vi "ExecuteMenuCommand.vi"(0 "reference":refnum<class "ClassNode.lvclass">, 1 "Command":string, 5 "error in (no error)":errorcluster) -> (14 "reference out":refnum<class "ClassNode.lvclass">, 15 "EditorAction":T3, 16 "FlattenCommandSettings":T1, 19 "error out":errorcluster)   [LabVIEW 2020, in "ClassNode.lvclass"]
uses:
  <resource>/Framework/Providers/Open_GDS/UML/ClassNode_class/ClassNode.lvclass
  <resource>/Framework/Providers/Open_GDS/UML/UMLEditor/UMLEditor EditorActionType.ctl
  <resource>/Framework/Providers/Open_GDS/UML/UMLEditor/UMLEditor FlattenCommandType.ctl
  <resource>/Framework/Providers/Open_GDS/UML/UMLEditor/UMLEditor ExecuteCommandType.ctl
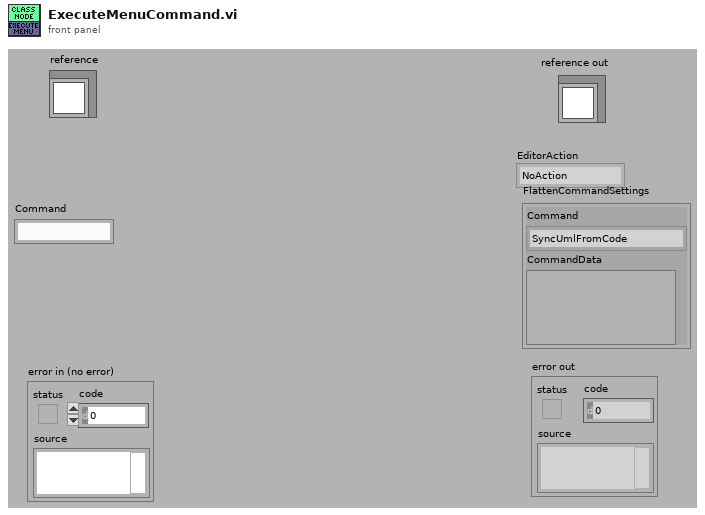
[diagram p1: front panel]
types:
  T1 = typedef "UMLEditor FlattenCommandType.ctl" = cluster{"Command":T2, "CommandData":variant}
  T2 = typedef "UMLEditor ExecuteCommandType.ctl" = enum16{"SyncUmlFromCode", "SyncCodeFromUML", "OpenClass", "OpenFile", "CreateClass", "CreateVI", "OpenClassAttribute", "LocateInProject", "GraphExecute"}
  T3 = typedef "UMLEditor EditorActionType.ctl" = enum16{"NoAction", "Repaint", "ExecuteCommand"}
  T4 = typedef "ClassNode.lvclass/ObjectAttributes.ctl" = cluster{"midHeight":dbl, "botHeight":dbl, "name":refnum<class "MultiLineString.lvclass">, "attributes":refnum<class "MultiLineString.lvclass">, "methods":refnum<class "MultiLineString.lvclass">, "DEFAULT_COMPARTMENT_HEIGHT":i32, "DEFAULT_WIDTH":i32, "DEFAULT_HEIGHT":i32, "showMethods":bool, "showAttributes":bool, "ClassPath":path}
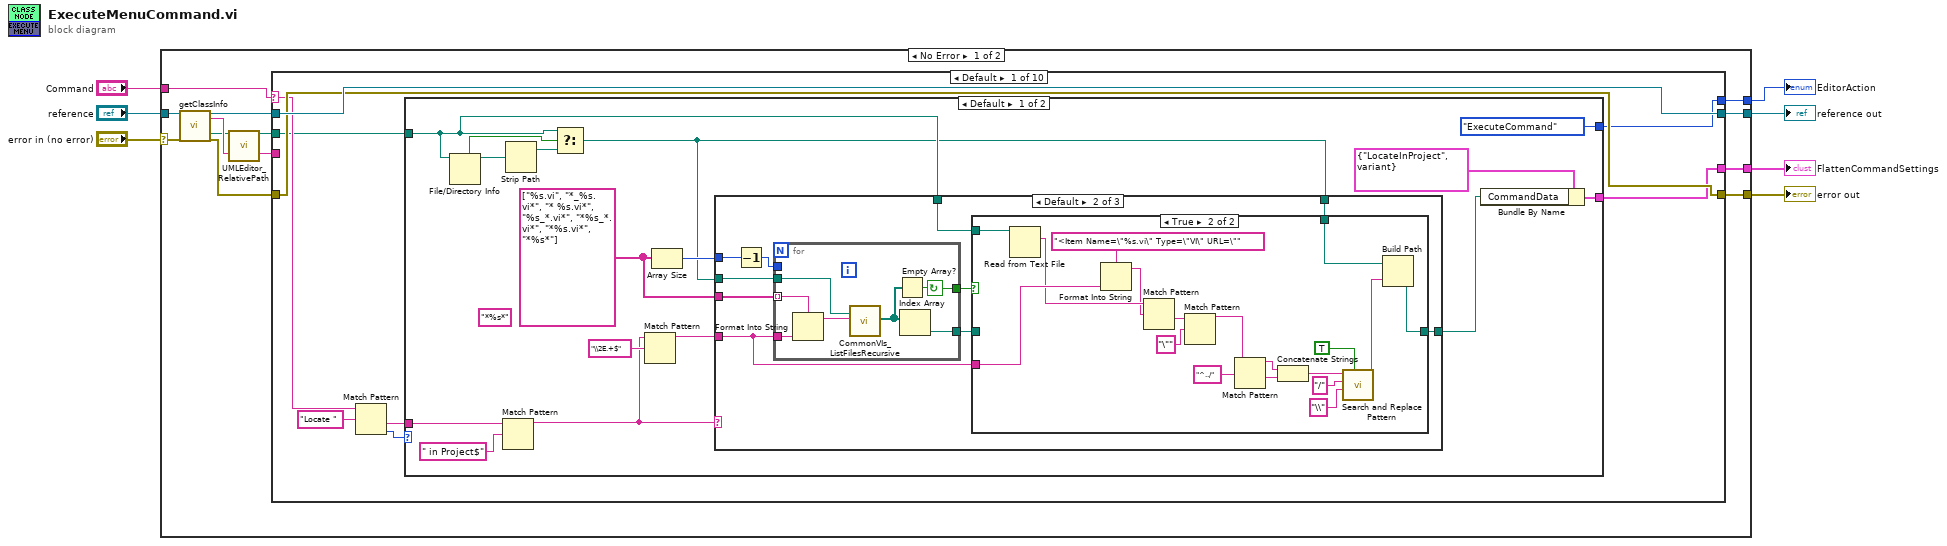
[diagram p0: block diagram]
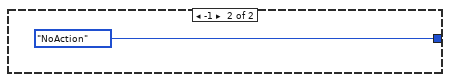
[diagram p5: hidden frame]
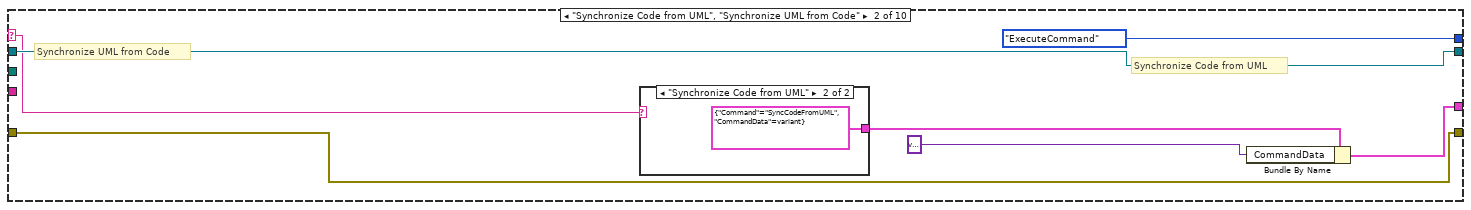
[diagram p6: hidden frame]
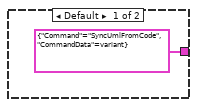
[diagram p7: hidden frame]
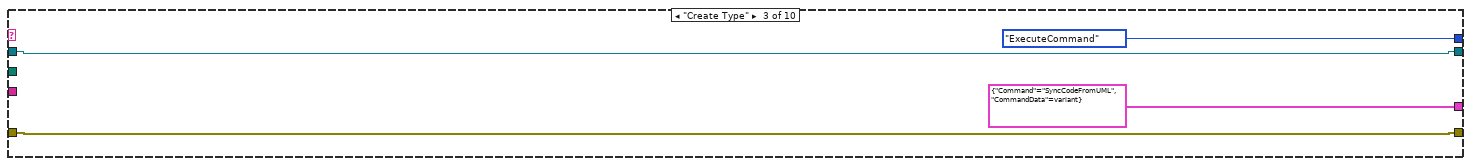
[diagram p8: hidden frame]
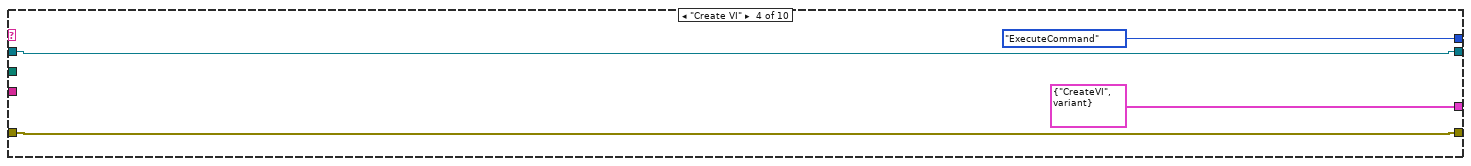
[diagram p9: hidden frame]
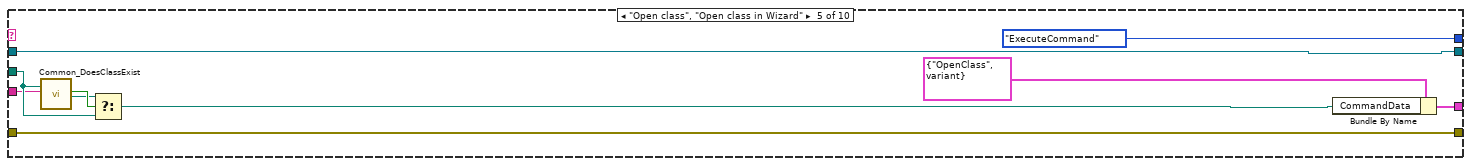
[diagram p10: hidden frame]
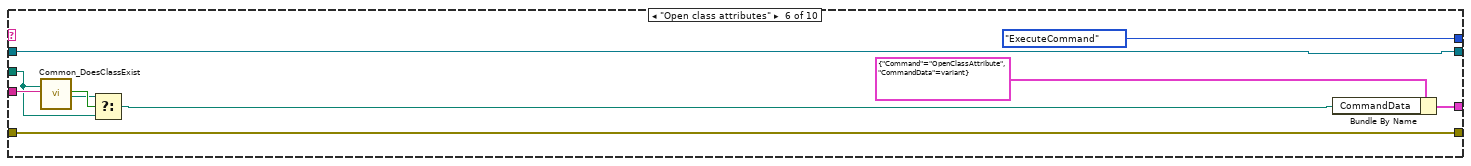
[diagram p11: hidden frame]
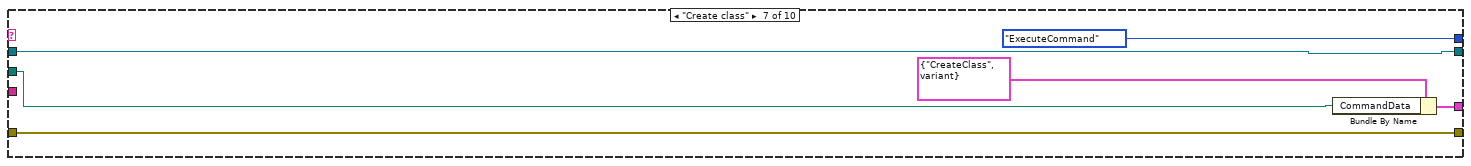
[diagram p12: hidden frame]
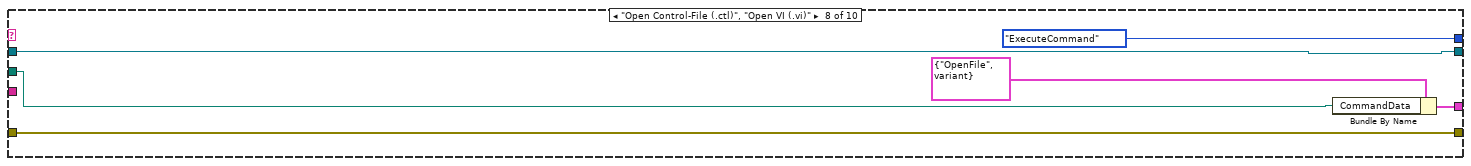
[diagram p13: hidden frame]
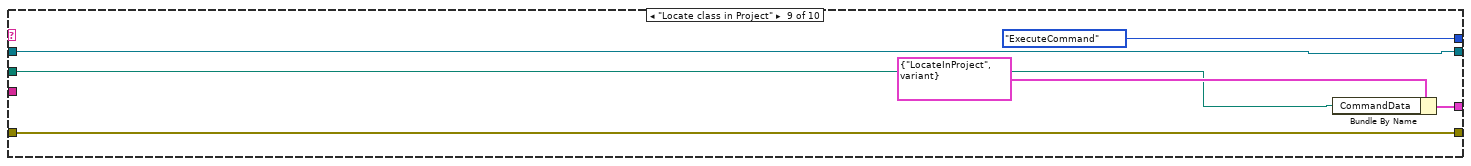
[diagram p14: hidden frame]
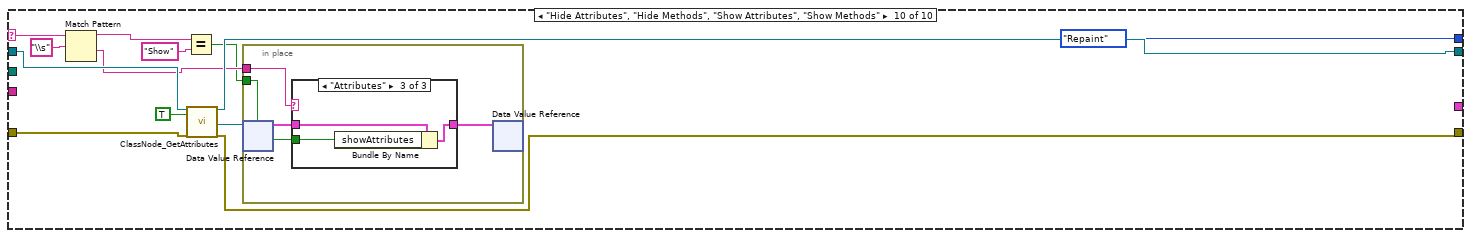
[diagram p15: hidden frame]
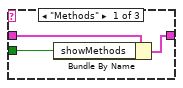
[diagram p16: hidden frame]
diagram:
  n1 = case shown="No Error" "error in (no error)" {
    selector: "error in (no error)" -> [w12 w162]
    tunnel: "reference" -> [w14 w163]
    tunnel: [w17 w162] -> w5
    tunnel: [w18 w163] -> w4
    tunnel: "Command" -> [w19 _]
    tunnel: [w16 _] -> w2
    tunnel: [w15 _] -> w1
    frame No Error {
      n2 = call-dynamic "getClassInfo.vi"("reference"=w14, "error in (no error)"=w12) -> ("reference out"=w13:refnum<class "ClassNode.lvclass">, "className"=w10:string, "ClassPath"=w9:path, "error out"=w11:errorcluster)  [unwired: 8 in, 6 out]
      n3 = call <resource>:"UMLEditor_RelativePath.vi"("Path In"=w9) -> ("ConvertToAbsolutePath(If possible)"=w8:path)  [unwired: 1 in, 17 out]
      n4 = case shown="Default" w19 {
        selector: w19 -> [w25 w83 _ _ _ _ _ _ _ w145]
        tunnel: w11 -> [w27 w87 w92 w96 w107 w110 w123 w129 w135 w147]
        tunnel: w13 -> [w28 w88 w93 w97 w108 w118 w124 w130 w136 w149]
        tunnel: [w28 w88 w93 w97 w108 w118 w124 w130 w136 w148] -> w18
        tunnel: [w27 w87 w92 w96 w107 w110 w123 w129 w135 w146] -> w17
        tunnel: [w26 UMLEditor_EditorActionType."ExecuteCommand" ("EditorAction") UMLEditor_EditorActionType."ExecuteCommand" ("EditorAction") UMLEditor_EditorActionType."ExecuteCommand" ("EditorAction") UMLEditor_EditorActionType."ExecuteCommand" ("EditorAction") UMLEditor_EditorActionType."ExecuteCommand" ("EditorAction") UMLEditor_EditorActionType."ExecuteCommand" ("EditorAction") UMLEditor_EditorActionType."ExecuteCommand" ("EditorAction") UMLEditor_EditorActionType."ExecuteCommand" ("EditorAction") UMLEditor_EditorActionType."Repaint" ("EditorAction")] -> w16
        tunnel: [w21 w85 T1 {"Command"=enum."SyncCodeFromUML", "CommandData"=variant} ("FlattenCommandSettings") T1 {"Command"=enum."CreateVI", "CommandData"=variant} ("FlattenCommandSettings") w105 w116 w121 w127 w133 _] -> w15
        tunnel: w8 -> [w20 _ _ _ w101 w111 w120 w126 w132 _]
        tunnel: w10 -> [_ _ _ _ w100 w112 _ _ _ _]
        frame Default {
          n5 = Match Pattern(string=w25, regular expression="Locate ") -> (after substring=w22:string, offset past match=w23:i32)  [unwired: 1 in, 2 out]
          n6 = case shown="Default" w23 {
            tunnel: [UMLEditor_EditorActionType."ExecuteCommand" ("EditorAction") UMLEditor_EditorActionType."NoAction" ("EditorAction")] -> w26
            tunnel: w22 -> [w44 _]
            tunnel: [w40 _] -> w21
            tunnel: w20 -> [w30 _]
            frame Default {
              (unwired) "*%s*" ("format string")
              w36 = string[] ["%s.vi", "*_%s.vi*", "* %s.vi*", "%s_*.vi*", "*%s_*.vi*", "*%s.vi*", "*%s*"]
              n7 = File/Directory Info(path=w30) -> (path out=w34:path, directory=w38:bool)  [unwired: 1 in, 5 out]
              n8 = Match Pattern(string=w44, regular expression=" in Project$") -> (before substring=w32:string)  [unwired: 1 in, 3 out]
              n9 = Strip Path(path=w34) -> (stripped path=w33:path)  [unwired: 1 out]
              n10 = Select(t=w30, s=w38, f=w33) -> (s? t:f=w29:path)
              n11 = Match Pattern(string=w32, regular expression="\\2E.+$") -> (before substring=w37:string)  [unwired: 4 out]
              n12 = Array Size(array=w36) -> (size(s)=w35:i32)
              n13 = case shown="Default" w32 {
                tunnel: [_ w48 w81] -> w31
                tunnel: w29 -> [_ w54 _]
                tunnel: w36 -> [_ w53 _]
                tunnel: w37 -> [_ w46 _]
                tunnel: w35 -> [_ w52 _]
                tunnel: w30 -> [_ w47 w81]
                tunnel: w29 -> [_ w45 _]
                frame "" {
                }
                frame Default {
                  n14 = Decrement(x=w52) -> (x-1=w51:i32)
                  n15 = for {
                    tunnel: w54 -> [w61]
                    tunnel: w53 -> [w60] mode=indexing
                    tunnel: w46 -> [w59]
                    tunnel: [w58] -> w49
                    tunnel: w51 -> [_]
                    tunnel: [w55] -> w50
                    stop <- w55 continue-if-true
                    n16 = Format Into String(format string=w60, w59) -> (resulting string=w56:string)  [unwired: 2 in, 1 out]
                    n17 = call <resource>:"CommonVIs_ListFilesRecursive.vi"("directory path"=w61, "FileSearchPattern"=w56) -> ("Files"=w57:path[])  [unwired: 4 in, 13 out]
                    n18 = Empty Array?(array=w57) -> (empty?=w55:bool)
                    n19 = Index Array(array=w57) -> (element=w58:path)  [unwired: 1 in]
                  }
                  n20 = case shown="True" w50 {
                    tunnel: w49 -> [w62 _]
                    tunnel: [w62 w63] -> w48
                    tunnel: w47 -> [_ w80]
                    tunnel: w46 -> [_ w78]
                    tunnel: w45 -> [_ w73]
                    frame False {
                    }
                    frame True {
                      n21 = Read from Text File(file (use dialog)=w80) -> (text=w77:string)  [unwired: 3 in, 3 out]
                      n22 = Format Into String(format string="<Item Name=\"%s.vi\" Type=\"VI\" URL=\"" ("regular expression"), w78) -> (resulting string=w76:string)  [unwired: 2 in, 1 out]
                      n23 = Match Pattern(string=w77, regular expression=w76) -> (after substring=w75:string)  [unwired: 1 in, 3 out]
                      n24 = Match Pattern(string=w75, regular expression="\"") -> (before substring=w65:string)  [unwired: 1 in, 3 out]
                      n25 = Match Pattern(string=w65, regular expression="^../") -> (before substring=w72:string, after substring=w71:string)  [unwired: 1 in, 2 out]
                      n26 = Concatenate Strings(w72, w71) -> (w70:string)
                      n27 = call <vilib>:"Search and Replace Pattern.vi"("string"=w70, "regular expression (\"\")"="/" ("regular expression (\"\")"), "replace string (\"\")"="\\" ("replace string (\"\")"), "replace all? (F)"=TRUE) -> ("result string"=w64:string)  [unwired: 1 in, 1 out]
                      n28 = Build Path(base path=w73, name or relative path=w64) -> (appended path=w63:path)
                    }
                  }
                }
                frame "item" {
                }
              }
              n29 = Bundle By Name(cluster=T1 {"Command"=enum."LocateInProject", "CommandData"=variant} ("FlattenCommandSettings"), "CommandData"=w31) -> (w40:T1)
            }
            frame -1 {
            }
          }
        }
        frame "Synchronize Code from UML", "Synchronize UML from Code" {
          # "Synchronize Code from UML"
          # "Synchronize UML from Code"
          n30 = case shown="\"Synchronize Code from UML\"" w83 {
            tunnel: [T1 {"Command"=enum."SyncUmlFromCode", "CommandData"=variant} ("FlattenCommandSettings") T1 {"Command"=enum."SyncCodeFromUML", "CommandData"=variant} ("FlattenCommandSettings")] -> w86
            frame Default {
            }
            frame "Synchronize Code from UML" {
            }
          }
          n31 = Bundle By Name(cluster=w86, "CommandData"=variant) -> (w85:T1)
        }
        frame "Create Type" {
        }
        frame "Create VI" {
        }
        frame "Open class", "Open class in Wizard" {
          n32 = call <resource>:"Common_DoesClassExist.vi"("ClassPath"=w101, "ClassName"=w100) -> ("llb-class"=w103:bool, "llb/LvCLass-Path"=w102:path)  [unwired: 16 out]
          n33 = Select(t=w102, s=w103, f=w101) -> (s? t:f=w104:path)
          n34 = Bundle By Name(cluster=T1 {"Command"=enum."OpenClass", "CommandData"=variant} ("FlattenCommandSettings"), "CommandData"=w104) -> (w105:T1)
        }
        frame "Open class attributes" {
          n35 = call <resource>:"Common_DoesClassExist.vi"("ClassPath"=w111, "ClassName"=w112) -> ("llb-class"=w114:bool, "llb/LvCLass-Path"=w113:path)  [unwired: 16 out]
          n36 = Select(t=w113, s=w114, f=w111) -> (s? t:f=w115:path)
          n37 = Bundle By Name(cluster=T1 {"Command"=enum."OpenClassAttribute", "CommandData"=variant} ("FlattenCommandSettings"), "CommandData"=w115) -> (w116:T1)
        }
        frame "Create class" {
          n38 = Bundle By Name(cluster=T1 {"Command"=enum."CreateClass", "CommandData"=variant} ("FlattenCommandSettings"), "CommandData"=w120) -> (w121:T1)
        }
        frame "Open Control-File (.ctl)", "Open VI (.vi)" {
          n39 = Bundle By Name(cluster=T1 {"Command"=enum."OpenFile", "CommandData"=variant} ("FlattenCommandSettings"), "CommandData"=w126) -> (w127:T1)
        }
        frame "Locate class in Project" {
          n40 = Bundle By Name(cluster=T1 {"Command"=enum."LocateInProject", "CommandData"=variant} ("FlattenCommandSettings"), "CommandData"=w132) -> (w133:T1)
        }
        frame "Hide Attributes", "Hide Methods", "Show Attributes", "Show Methods" {
          n41 = Match Pattern(string=w145, regular expression="\\s") -> (before substring=w141:string, after substring=w139:string)  [unwired: 3 out]
          n42 = Equal?(x=w141, y="Show") -> (x = y?=w138:bool)
          n43 = call <resource>:"ClassNode_GetAttributes.vi"("reference in"=w149, "OnlyGetDvrReference(False)"=TRUE, "error in (no error)"=w147) -> ("reference out"=w148:refnum<class "ClassNode.lvclass">, "DataRef"=w140:refnum<data-value>, "error out"=w146:errorcluster)  [unwired: 13 in, 1 out]
          n44 = in-place {
            in-place-border: w139 -> [w154]
            in-place-border: w138 -> [w152]
            n45 = in-place-dvr #1(w140) -> (w153:T4)  [unwired: 1 out]
            n46 = case shown="\"Attributes\"" w154 {
              tunnel: w153 -> [w157 w158 w161]
              tunnel: [w156 w158 w160] -> w151
              tunnel: w152 -> [w155 _ w159]
              frame "Methods" {
                n47 = Bundle By Name(cluster=w157, "showMethods"=w155) -> (w156:T4)
              }
              frame Default {
              }
              frame "Attributes" {
                n48 = Bundle By Name(cluster=w161, "showAttributes"=w159) -> (w160:T4)
              }
            }
            n49 = in-place-dvr #1(w151) -> ()  [unwired: 2 out]
          }
        }
      }
    }
    frame Error {
    }
  }
  "reference out" <- w4
  "error out" <- w5
  "FlattenCommandSettings" <- w1
  "EditorAction" <- w2
